vi "MakeArrayTD (Variant).vi"(8 "error in (no error)":errorcluster, 10 "rank":i16, 11 "Element type_id":variant) -> (0 "error out":errorcluster, 2 "Default Data":string, 3 "td":i16[](array[numeric]) format="%.0x")   [LabVIEW 2017]
uses:
  <userlib>/_OpenG.lib/lvdata/lvdata.llb/Type Descriptor Enumeration__ogtk.ctl
panel:
  # "LVHDF5 Toolkit\nCopyright (c) 2005-2013 by Jason D. Sommerville\nCopyright (c) 2014 by UPVI, LLC.\n\nThis use and distribution of this file is governed by the terms found in \nLICENSE.txt distributed with this toolkit and installed at\n <user.lib>\\_lvhdf5\\LICENSE.txt"
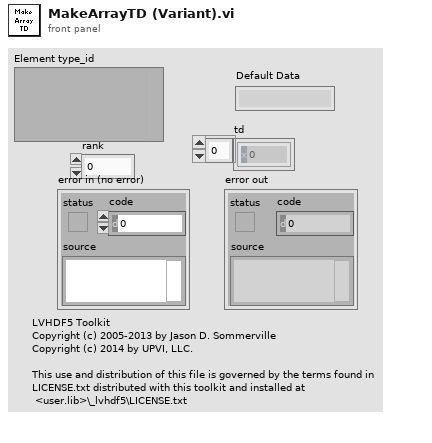
[diagram p1: front panel]
types:
  T1 = typedef "Type Descriptor Enumeration__ogtk.ctl" = enum8{"<Null>", "I8", "I16", "I32", "I64", "U8", "U16", "U32", "U64", "SGL", "DBL", "EXT", "CSG", "CDB", "CXT", "0x0F", "0x10", "0x11", "0x12", "0x13", "0x14", "Enum U8", "Enum U16", "Enum U32", "Enum U64", "SGL PQ", "DBL PQ", "EXT PQ", "CSG PQ", "CDB PQ", "CXT PQ", "0x1F", "0x20", "Boolean", "0x22", "0x23", "0x24", "0x25", "0x26", "0x27", "0x28", "0x29", "0x2A", "0x2B", "0x2C", "0x2D", "0x2E", "0x2F", "String", "0x31", "Path", "Pict", "0x34", "0x35", "0x36", "DAQ", "0x38", "0x39", "0x3A", "0x3B", "0x3C", "0x3D", "0x3E", "0x3F", "Array", "0x41", "0x42", "0x43", "0x44", "0x45", "0x46", "0x47", "0x48", "0x49", "0x4A", "0x4B", "0x4C", "0x4D", "0x4E", "0x4F", "Cluster", "0x51", "0x52", "Variant", "Waveform", "0x55", "0x56", "0x57", "0x58", "0x59", "0x5A", "0x5B", "0x5C", "0x5D", "0x5E", "0x5F", "0x60", "0x61", "0x62", "0x63", "0x64", "0x65", "0x66", "0x67", "0x68", "0x69", "0x6A", "0x6B", "0x6C", "0x6D", "0x6E", "0x6F", "Refnum"}
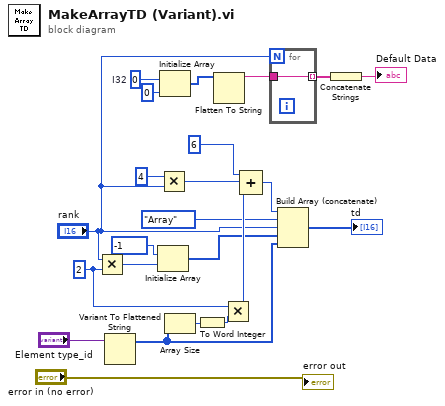
[diagram p0: block diagram]
diagram:
  w2 = 0  # I32
  w17 = i16 2 ("y")
  n1 = Multiply(x="rank", y=w17) -> (x*y=w13:i16)
  n2 = Variant To Flattened String(Variant="Element type_id") -> (1:w6:i16[])  [unwired: 1 out]
  n3 = Initialize Array(i16 -1 ("y"), w13) -> (w15:i16[])
  n4 = Multiply(x=i16 4, y="rank") -> (x*y=w19:i16)
  n5 = Initialize Array(w2, 0 ("dimension size")) -> (w4:i32[])
  n6 = Array Size(array=w6) -> (size(s)=w16:i32)
  n7 = To Word Integer(number=w16) -> (16bit integer=w21:i16)
  n8 = Flatten To String(anything=w4) -> (data string=w1:string)  [unwired: 3 in, 2 out]
  n9 = Multiply(x=w17, y=w21) -> (x*y=w20:i16)
  n10 = Compound Arithmetic op=ADD(i16 6, w19, w20) -> (w22:i16)
  n11 = for {
    N: "rank" -> [_]
    tunnel: [w24] -> w10 mode=indexing
    tunnel: w1 -> [w24]
  }
  n12 = Build Array (concatenate)(w22, Type_Descriptor_Enumeration__ogtk."Array" ("Type Descriptor Enumeration"), "rank", w15, w6) -> (→"td":i16[])
  n13 = Concatenate Strings(w10) -> (→"Default Data":string)
  "error out" <- "error in (no error)"
